vi "Global 1.vi"() -> ()   [LabVIEW 2013]
panel:
  out "isRun":bool
  out "Y":dbl
  out "X":dbl
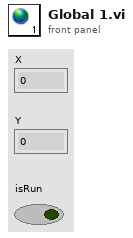
[diagram p1: front panel]
diagram:
